vi "Pose3d_Times.vi"(9 "Scalar":dbl, 11 "in Pose3d":T1={"Translation3d"={"X"=0.0, "Y"=0.0, "Z"=0.0}, "Rotation3d"={"Q_quaternion"={"R"=1.0, "V"=[0.0, 0.0, 0.0]}}} {"Translation3d"."Z" format="%14.3f"; "Translation3d"."Y" format="%14.3f"; "Translation3d"."X" format="%14.3f"}) -> (3 "out Pose3d":T1={"Translation3d"={"X"=0.0, "Y"=0.0, "Z"=0.0}, "Rotation3d"={"Q_quaternion"={"R"=1.0, "V"=[0.0, 0.0, 0.0]}}} {"Translation3d"."Z" format="%14.3f"; "Translation3d"."Y" format="%14.3f"; "Translation3d"."X" format="%14.3f"})   [LabVIEW 2019, in "Trajectory_Library.lvlib"]
doc: "Multiply the pose by the given scalar and returns the new pose3d. \n\nParameters:\n - IN POSE3D - The input POSE data structure\n - Scalar - The value to multiply the pose by.\n\nReturn:\n - OUT POSE3D - The output pose."
uses:
  TypeDef/POSE3D.ctl
  TypeDef/TRANSLATION3D.ctl
  TypeDef/ROTATION3D.ctl
  TypeDef/QUATERNION.ctl
  Transform3d_GetTranslation3d.vi
  Transform3d_GetRotation3d.vi
  Translation3d_Plus.vi
  Translation3d_RotateBy.vi
  Rotation3d_Plus.vi
  Translation3d_Create.vi
  Rotation3d_GetQuaterion.vi
  Quaternion_New.vi
  Quaternion_Times.vi
  Quaternion_Inverse.vi
  Quaternion_Get_All.vi
  Rotation3d_RotateBy.vi
  Rotation3d_Create_Quaternion.vi
  Quaternion_Normalize.vi
  Quaternion_New_Default.vi
  Trajectory_Library.lvlib
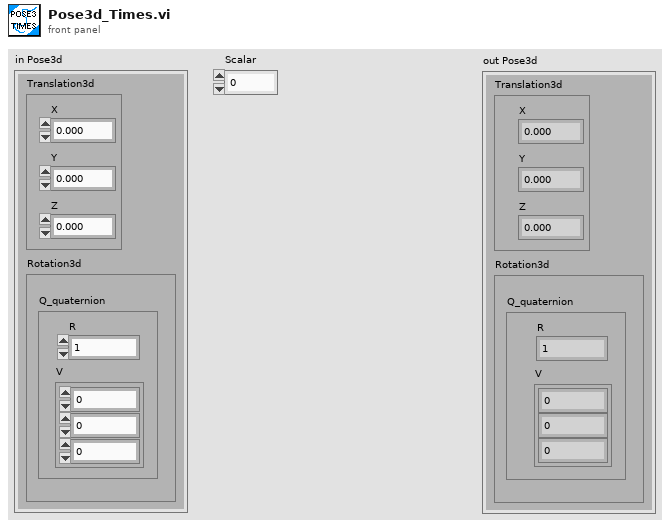
[diagram p1: front panel]
types:
  T1 = typedef "Trajectory_Library.lvlib/POSE3D.ctl" = cluster{"Translation3d":T2, "Rotation3d":T3}
  T2 = typedef "Trajectory_Library.lvlib/TRANSLATION3D.ctl" = cluster{"X":dbl, "Y":dbl, "Z":dbl}
  T3 = typedef "Trajectory_Library.lvlib/ROTATION3D.ctl" = cluster{"Q_quaternion":T4}
  T4 = typedef "Trajectory_Library.lvlib/QUATERNION.ctl" = cluster{"R":dbl, "V":dbl[]}
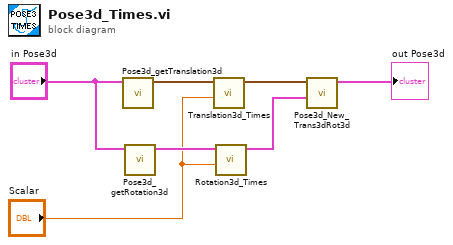
[diagram p0: block diagram]
diagram:
  n1 = call "Pose3d_getTranslation3d.vi"("in Pose3d"="in Pose3d") -> ("out Translation3d"=w7:T2)  [unwired: 10 in]
  n2 = call "Pose3d_getRotation3d.vi"("in Pose3d"="in Pose3d") -> ("out Rotation3d"=w5:T3)  [unwired: 10 in]
  n3 = call "Translation3d_Times.vi"("Scalar"="Scalar", "In Translation3d"=w7) -> ("Out Translation3d"=w4:T2)  [unwired: 9 in]
  n4 = call "Rotation3d_Times.vi"("Scalar"="Scalar", "in Rotation3d"=w5) -> ("out Rotation3d"=w3:T3)  [unwired: 9 in]
  n5 = call "Pose3d_New_Trans3dRot3d.vi"("Rotation3d"=w3, "Translation3d"=w4) -> ("outPose3d"=→"out Pose3d":T1)  [unwired: 9 in]
